vi "SpectralMeasurementsSubVI.vi"(0 "Signals":waveform(dbl)[](array[waveform]), 2 "Restart Averaging":bool, 7 "error in (no error)":errorcluster, 12 "Spectrum Averaging Parameters":T2={"averaging mode"=1, "weighting mode"=0, "number of averages"=2} {"averaging mode" items=["No averaging", "Vector averaging", "RMS averaging", "Peak hold"]; "weighting mode" items=["Linear", "Exponential"]}, 13 "View":T1) -> (8 "FFT - (RMS)":cluster{"f0":dbl, "df":dbl, "magnitude":dbl[]}[](array[cluster]), 9 "averaging done":bool, 10 "Phase":cluster{"f0":dbl, "df":dbl, "phase":dbl[]}[](array[cluster]), 11 "error out":errorcluster)   [LabVIEW 2022 SP3]
uses:
  <vilib>/express/express analysis/Spectral/Block/exnSpectralBlock spectral measurements RMS array WFM.vi
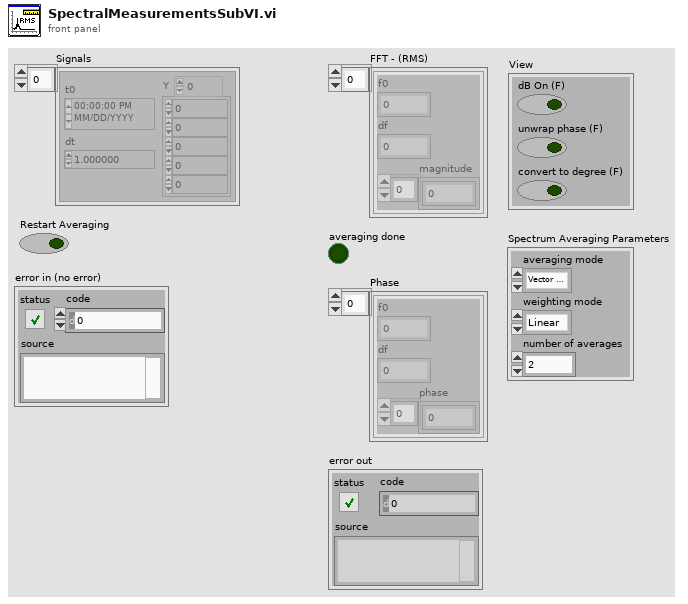
[diagram p1: front panel]
types:
  T1 = cluster{"dB On (F)":bool, "unwrap phase (F)":bool, "convert to degree (F)":bool}
  T2 = cluster{"averaging mode":u16, "weighting mode":u16, "number of averages":u32}
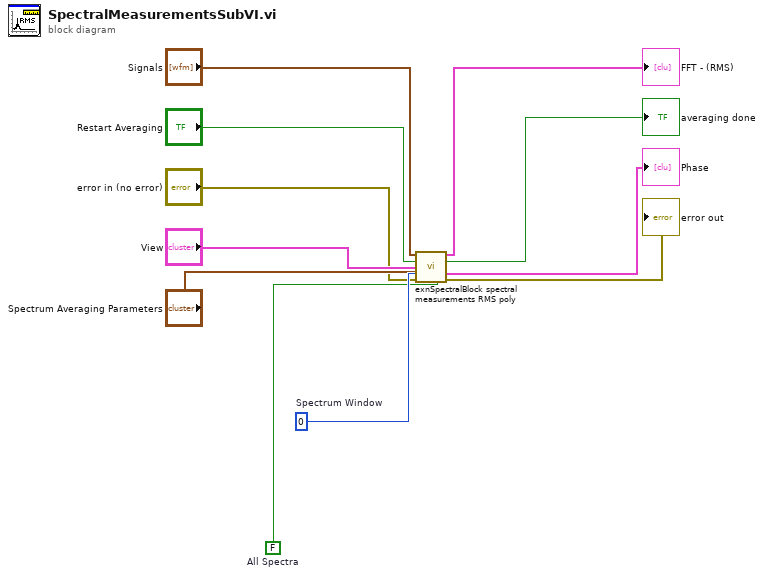
[diagram p0: block diagram]
diagram:
  w7 = FALSE  # All Spectra
  w9 = u16 0  # Spectrum Window
  n1 = call-poly <vilib>:"exnSpectralBlock spectral measurements RMS poly.vi"("Signals"="Signals", "Restart Averaging"="Restart Averaging", "View"="View", "Spectrum Window"=w9, "error in (no error)"="error in (no error)", "Spectrum Averaging Parameters"="Spectrum Averaging Parameters", "All Spectra"=w7) -> ("Measurement Output"=→"FFT - (RMS)":cluster{"f0":dbl, "df":dbl, "magnitude":dbl[]}[], "averaging done"=→"averaging done":bool, "Phase"=→"Phase":cluster{"f0":dbl, "df":dbl, "phase":dbl[]}[], "error out"=→"error out":errorcluster)  [unwired: 5 in]
